vi "SSL Detection Frame Robots Estimator.vi"(5 "Time Stamp":timestamp, 7 "Life Time":dbl=1.0, 10 "dt":dbl, 11 "Robots":T1[](array[typedef]) {"height" format="%+4.3f"; "pixel_y" format="%+4.3f"; "pixel_x" format="%+4.3f"; "orientation" format="%+4.3f"; "y" format="%+4.3f"; "confidence" format="%4.3f"; "x" format="%+4.3f"}) -> (3 "Est. Robots":T1[](array[typedef]) {"height" format="%+4.3f"; "pixel_y" format="%+4.3f"; "pixel_x" format="%+4.3f"; "orientation" format="%+4.3f"; "y" format="%+4.3f"; "confidence" format="%4.3f"; "x" format="%+4.3f"})   [LabVIEW 2018]
uses:
  SSL Detection Robot.ctl
  <vilib>/Analysis/Matrix/Datatypes/RealMatrix.ctl
  <vilib>/Analysis/Matrix/NI_Matrix.lvlib
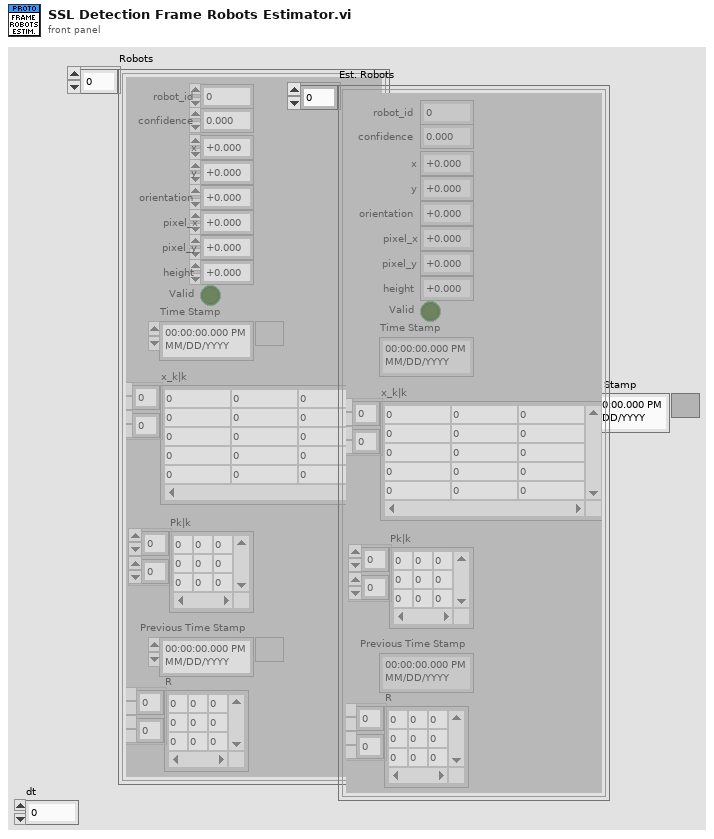
[diagram p1: front panel]
types:
  T1 = typedef "SSL Detection Robot.ctl" = cluster{"x":sgl, "robot_id":u32, "confidence":sgl, "y":sgl, "orientation":sgl, "pixel_x":sgl, "pixel_y":sgl, "height":sgl, "Valid":bool, "Time Stamp":timestamp, "x_k|k":T2, "Pk|k":T2, "Previous Time Stamp":timestamp, "R":T2}
  T2 = typedef "NI_Matrix.lvlib/RealMatrix.ctl" = dbl[][]
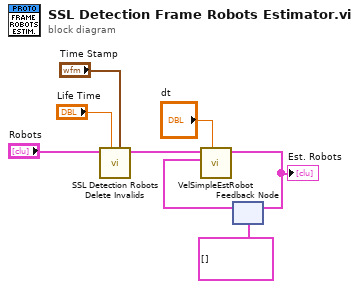
[diagram p0: block diagram]
diagram:
  n1 = call "SSL Detection Robots Delete Invalids.vi"("Now"="Time Stamp", "Life Time"="Life Time", "Robots In"="Robots") -> ("Robots Out"=w5:T1[])  [unwired: 8 in]
  n2 = feedback #1(T1[] []) -> (w3:T1[])
  n3 = call "VelSimpleEstRobot.vi"("dt"="dt", "Array in"=w3, "Robots Out"=w5) -> ("Array out"=w4:T1[])  [unwired: 8 in]
  "Est. Robots" <- w4
  n4 = feedback-in #1(w4) -> ()
